vi "T3AWG Open.vi"(8 "error in (no error)":errorcluster, 10 "Reset (True)":bool=TRUE, 11 "t3awg":T1 {"t3awg fs rules"."fs-step [Hz]" format="%#_6p"; "t3awg fs rules"."fs-max [Hz]" format="%#_6p"; "t3awg fs rules"."for f0 <" format="%#_6p"; "t3awg fs rules"."fs-min [Hz]" format="%#_6p"}) -> (0 "error out":errorcluster, 2 "idn string":string, 3 "t3awg out":T1 {"t3awg fs rules"."fs-step [Hz]" format="%#_6p"; "t3awg fs rules"."fs-max [Hz]" format="%#_6p"; "t3awg fs rules"."for f0 <" format="%#_6p"; "t3awg fs rules"."fs-min [Hz]" format="%#_6p"})   [LabVIEW 2020, in "Active Technologies AWG3000.lvlib"]
uses:
  Active Technologies AWG3000.lvlib
  T3AWG Session.ctl
  T3AWG Load Z.ctl
  fgen_ramdac_fs_rules.ctl
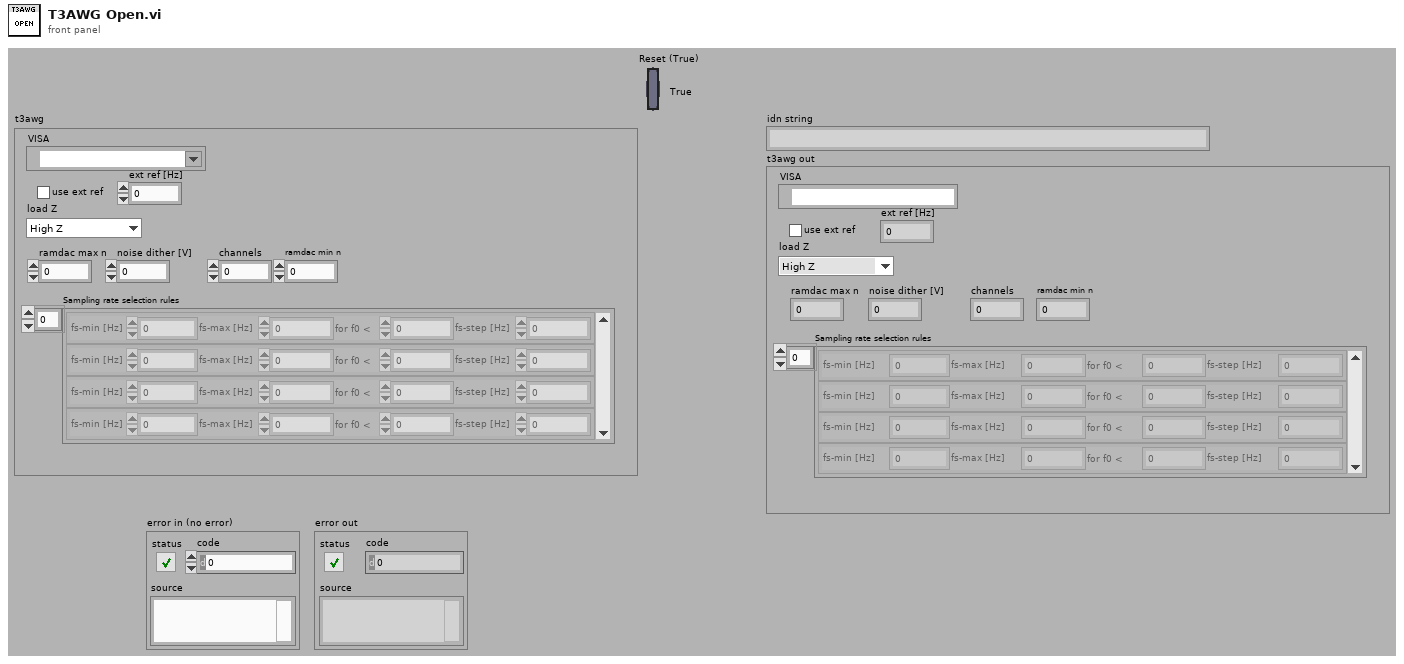
[diagram p1: front panel]
types:
  T1 = typedef "Active Technologies AWG3000.lvlib/T3AWG Session.ctl" = cluster{"VISA":refnum<visa-resource-name>, "use ext ref":bool, "ext ref [Hz]":dbl, "load Z":T2, "ramdac max n":i32, "noise dither [V]":dbl, "t3awg fs rules":T3[], "channels":i32, "ramdac min n":i32}
  T2 = typedef "Active Technologies AWG3000.lvlib/T3AWG Load Z.ctl" = enum16{"High Z", "50 Ohm"}
  T3 = typedef "Active Technologies AWG3000.lvlib/fgen_ramdac_fs_rules.ctl" = cluster{"fs-min [Hz]":dbl, "fs-max [Hz]":dbl, "for f0 < ":dbl, "fs-step [Hz]":dbl}
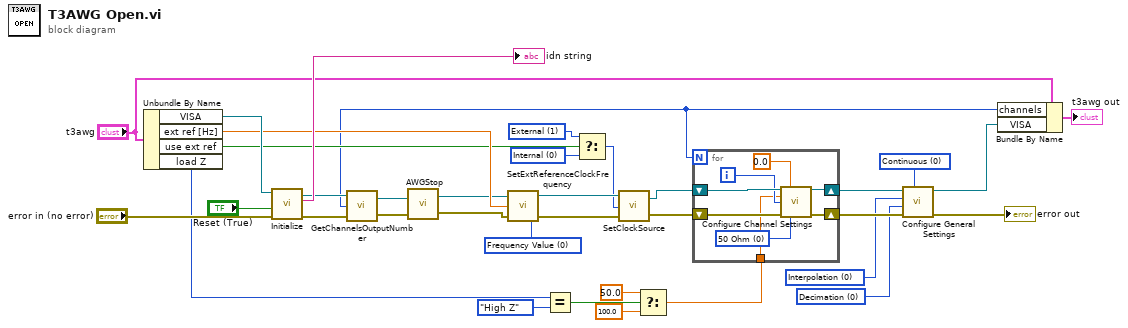
[diagram p0: block diagram]
diagram:
  w12 = u16 0 items=["Decimation", "Cut Tail", "Cut Head"] ("Sample Decreasing Startegy")
  w13 = u16 0 items=["Interpolation", "Return Zero", "Hold Last", "Samples Multiplication"] ("Sample Increasing Startegy")
  w14 = u16 0 items=["Continuous", "Single/Burst", "Triggered Continuous", "Stepped", "Advanced"] ("Run Mode")
  w24 = u16 0 items=["Frequency Value", "Default", "Minimum", "Maximum"] ("External  Reference Clock Option")
  w27 = u16 1 items=["Internal", "External"] ("Clock Source")
  w28 = u16 0 items=["Internal", "External"] ("Clock Source")
  n1 = Unbundle By Name("t3awg") -> ("VISA"=w35:refnum<visa-resource-name>, "ext ref [Hz]"=w33:dbl, "use ext ref"=w29:bool, "load Z"=w10:T2)
  n2 = call "Initialize.vi"("error in (no error)"="error in (no error)", "Reset (True)"="Reset (True)", "VISA resource name"=w35) -> ("error out"=w6:errorcluster, "idn string"=→"idn string":string, "VISA resource name out"=w3:refnum<visa-resource-name>)  [unwired: 3 in, 3 out]
  n3 = call "GetChannelsOutputNumber.vi"("error in (no error)"=w6, "VISA resource name"=w3) -> ("error out"=w5:errorcluster, "VISA resource name out"=w4:refnum<visa-resource-name>, "Output Channels Number"=w2:i8)
  n4 = call "AWGStop.vi"("error in (no error)"=w5, "VISA resource name"=w4) -> ("error out"=w18:errorcluster, "VISA resource name out"=w19:refnum<visa-resource-name>)
  n5 = call "SetExtReferenceClockFrequency.vi"("External  Reference Clock Option"=w24, "error in (no error)"=w18, "External Reference Clock (Hz)"=w33, "VISA resource name"=w19) -> ("error out"=w32:errorcluster, "VISA resource name out"=w31:refnum<visa-resource-name>)
  n6 = Equal?(x=w10, y=T3AWG_Load_Z."High Z") -> (x = y?=w8:bool)
  n7 = Select(t=w27, s=w29, f=w28) -> (s? t:f=w30:u16)
  n8 = call "SetClockSource.vi"("error in (no error)"=w32, "Clock Source"=w30, "VISA resource name"=w31) -> ("error out"=w22:errorcluster, "VISA resource name out"=w21:refnum<visa-resource-name>)
  n9 = Select(t=50.0, s=w8, f=100.0) -> (s? t:f=w11:dbl)
  n10 = for {
    N: w2 -> [_]
    shift-right: [w42] -> w20
    shift-left: w22 -> [w44]
    shift-right: [w41] -> w17
    shift-left: w21 -> [w43]
    tunnel: w11 -> [w39]
    i -> [w40]
    w38 = u8 0 items=["50 Ohm", "Low"] ("Output Impedance")
    n11 = call "Configure Channel Settings.vi"("VISA resource name"=w43, "Base Line Offset (V)"=0.0, "Amplitude Scale (%)"=w39, "Channel (0: Channel 1)"=w40, "error in (no error)"=w44, "Output Impedance"=w38) -> ("VISA resource name out"=w41:refnum<visa-resource-name>, "error out"=w42:errorcluster)  [unwired: 8 in]
  }
  n12 = call "Configure General Settings.vi"("Run Mode"=w14, "error in (no error)"=w20, "Sample Decreasing Startegy"=w12, "Sample Increasing Startegy"=w13, "VISA resource name"=w17) -> ("error out"=→"error out":errorcluster, "VISA resource name out"=w15:refnum<visa-resource-name>)  [unwired: 4 in]
  n13 = Bundle By Name(cluster="t3awg", "channels"=w2, "VISA"=w15) -> (→"t3awg out":T1)
